vi "Chasis _Omni_Basic.vi"   [LabVIEW 2012, in "Fiel Orientation Compass.lvrbt"]
uses:
  Fiel Orientation Compass.lvrbt
  <vilib>/NXT/Subs/LVHSConnector.ctl
  <vilib>/NXT/NXTIO Xnodes/NXTIOXNode/NXTIO.xnode
  <vilib>/NXT/NXTIO Xnodes/NXTIONodeSubVIs/TETRIX IO Move DC Motors.vi
  <vilib>/NXT/NXTIO Xnodes/AddressXNode/NXTIOAddress.xnode
  <vilib>/FTC/FTC Interpret Motor Power From Left X Axis.vi
  <vilib>/FTC/FTC Interpret Motor Power From Left Y Axis.vi
  <vilib>/FTC/FTC Interpret Motor Power From Right X Axis.vi
  <vilib>/NXT/Dual Mode Library/prims/inRangeAndCoerce/inRangeAndCoerce_int.vi
  <vilib>/NXT/LegoClasses/BrickReference/BrickReference.lvclass
  <vilib>/NXT/Hardware/Plugins/Tetrix DC Motor/TetrixDCMotorAddress.ctl
panel:
  # "This VI was generated based on your configuration in the Remote Control Editor. You may modify the code as needed for your robot. To test this program for an FTC match, return to the Remote Control Editor, select the \"Run Program\" tab, and choose \"FTC Game\"."
types:
  T1 = typedef "LVHSConnector.ctl" = refnum<class "BrickReference.lvclass">
  T2 = typedef "FTC ControllerState.ctl" = cluster{"Left X":i8, "Left Y":i8, "Right X":i8, "Right Y":i8, "Button Encoding 9-12":u8, "Button Encoding 1-8":u8, "POV":T3}
  T3 = typedef "FTC POVState.ctl" = i8
  T4 = typedef "FTC ButtonEventType.ctl" = enum16{"Pressed", "Released"}
  T5 = cluster{"Button ID":enum16{"None", "Button 1", "Button 2", "Button 3", "Button 4", "Button 5", "Button 6", "Button 7", "Button 8", "Button 9", "Button 10", "Button 11", "Button 12", "POV Up", "POV Up Right", "POV Right", "POV Down Right", "POV Down", "POV Down Left", "POV Left", "POV Up Left"}, "Event Type":T4}[]
  T6 = enum16{"None", "Button 1", "Button 2", "Button 3", "Button 4", "Button 5", "Button 6", "Button 7", "Button 8", "Button 9", "Button 10", "Button 11", "Button 12", "POV Up", "POV Up Right", "POV Right", "POV Down Right", "POV Down", "POV Down Left", "POV Left", "POV Up Left"}
  T7 = typedef "TetrixDCMotorAddress.ctl" = i16
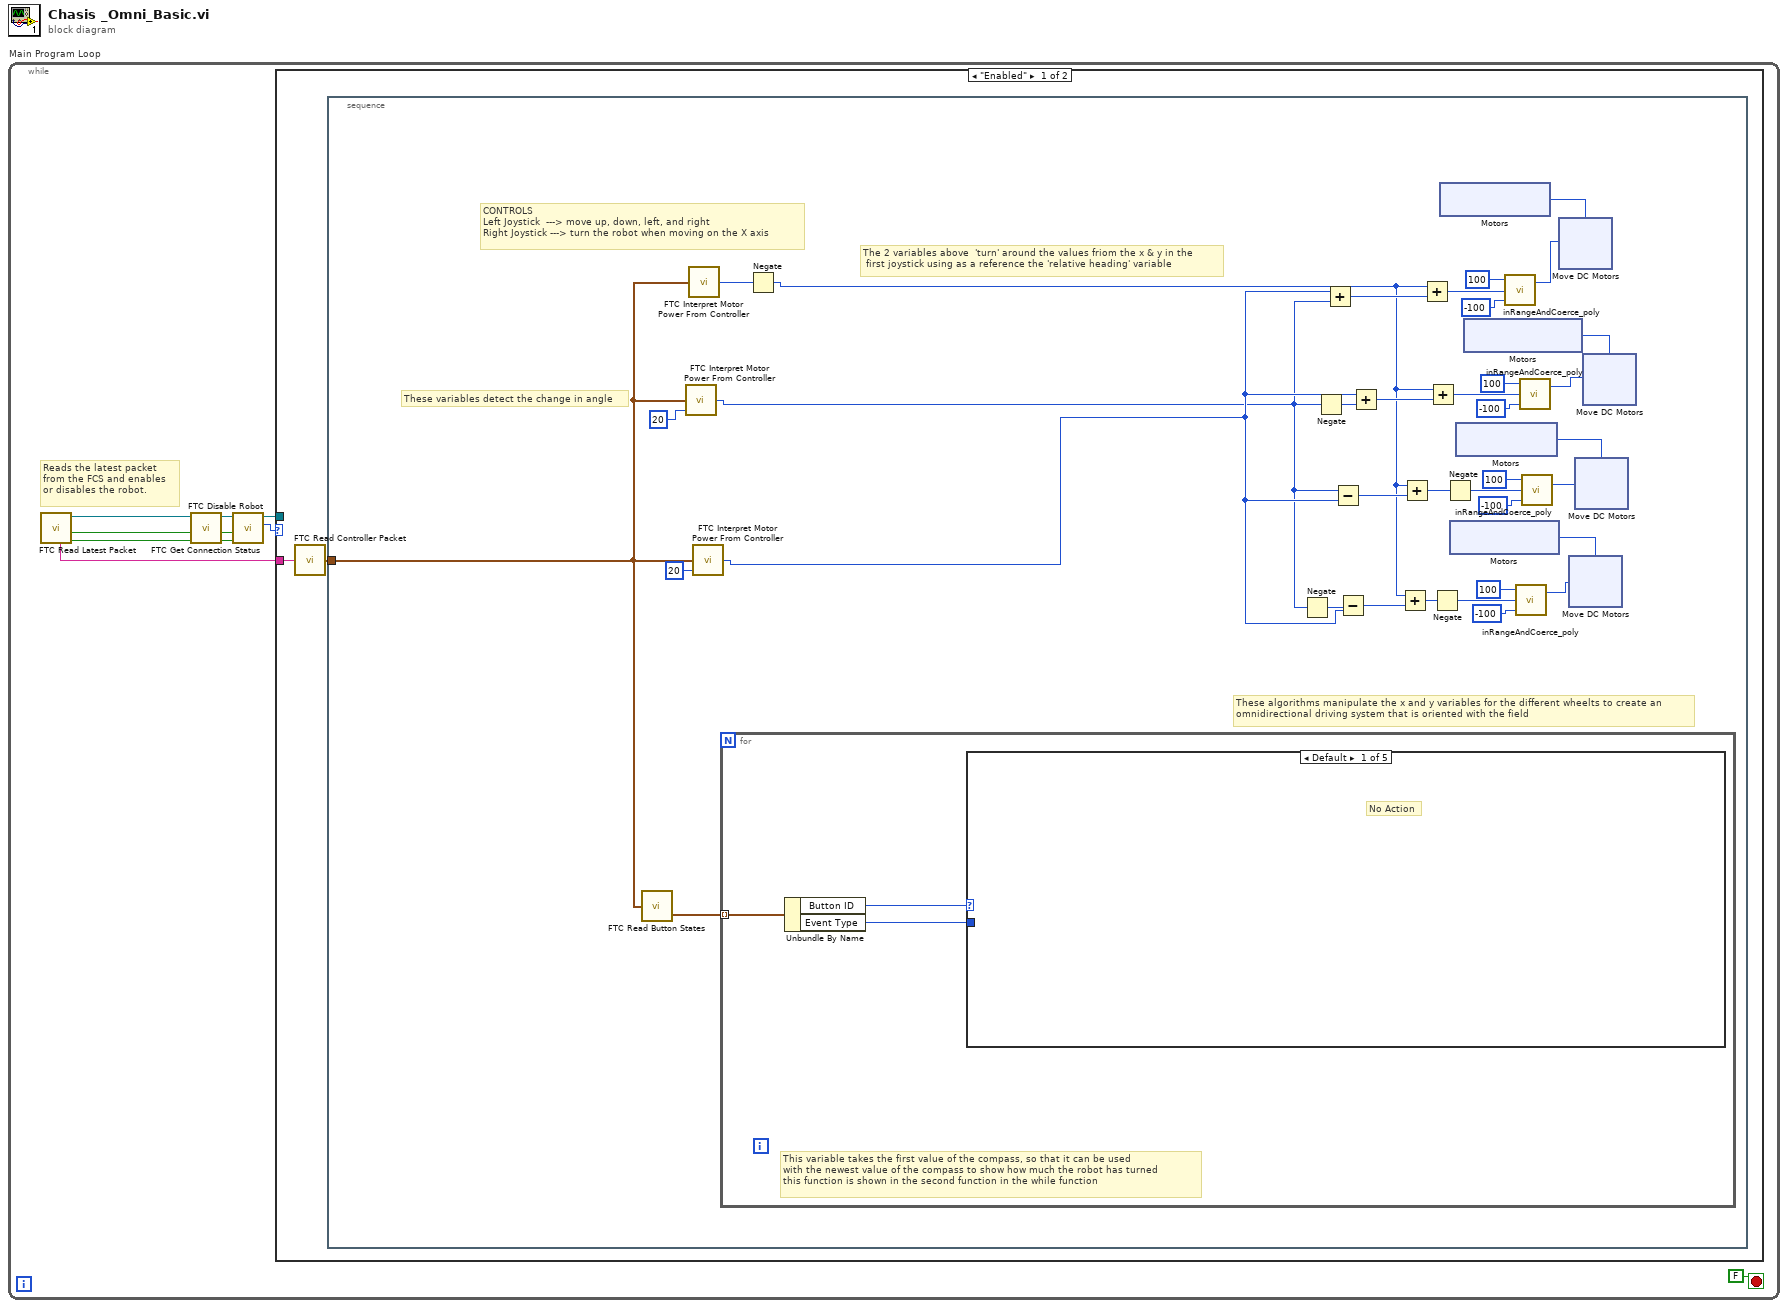
[diagram p0: block diagram]
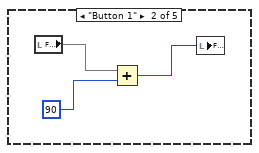
[diagram p2: hidden frame]
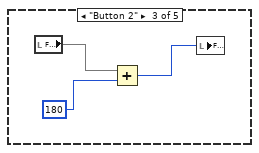
[diagram p3: hidden frame]
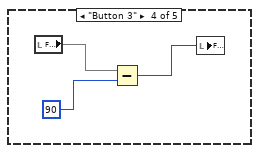
[diagram p4: hidden frame]
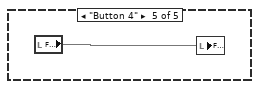
[diagram p5: hidden frame]
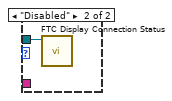
[diagram p6: hidden frame]
diagram:
  n1 = while "Main Program Loop" {
    stop <- FALSE stop-if-true
    # "Reads the latest packet\nfrom the FCS and enables\nor disables the robot."
    n2 = call <vilib>:"FTC Read Latest Packet.vi"() -> ("Packet Received?"=w8:bool, "Stopped?"=w5:bool, "NXT"=w7:T1, "Controller 1"=w9:string)  [unwired: 6 in, 2 out]
    n3 = call <vilib>:"FTC Get Connection Status.vi"("Packet Received?"=w8, "Stopped?"=w5, "NXT"=w7) -> ("Online?"=w2:bool, "Stopped?"=w3:bool, "NXT"=w4:T1)  [unwired: 5 in]
    n4 = call <vilib>:"FTC Disable Robot.vi"("Online?"=w2, "Stopped?"=w3, "NXT"=w4) -> ("Enabled?"=w6:enum16{"Disabled", "Enabled"}, "NXT"=w1:T1)  [unwired: 3 in]
    n5 = case "disableCase" shown="\"Enabled\"" w6 {
      tunnel: w9 -> [w12 _]
      tunnel: w1 -> [_ w94]
      frame "Enabled" {
        n6 = call <vilib>:"FTC Read Controller Packet.vi"("Packet"=w12) -> ("Controller State"=w11:T2)  [unwired: 4 in]
        n7 = stacked-sequence "controller1Actions" {
          tunnel: w11 -> [w48]
          frame #0 {
            # "These algorithms manipulate the x and y variables for the different wheelts to create an\nomnidirectional driving system that is oriented with the field"
            # "The 2 variables above  'turn' around the values friom the x & y in the\n\tfirst joystick using as a reference the 'relative heading' variable"
            # "These variables detect the change in angle"
            # "CONTROLS\nLeft Joystick  ---> move up, down, left, and right                   \nRight Joystick ---> turn the robot when moving on the X axis"
            n8 = call <vilib>:"FTC Read Button States.vi"("Controller State"=w48) -> ("Button Events"=w47:T5)  [unwired: 2 in, 1 out]
            n9 = call-poly <vilib>:"FTC Interpret Motor Power From Controller.vi"("Deadband (10)"=i8 20, "Controller State"=w48) -> ("Power"=w14:i8)  [unwired: 1 in]
            n10 = call-poly <vilib>:"FTC Interpret Motor Power From Controller.vi"("Controller State"=w48) -> ("Power"=w46:i8)  [unwired: 2 in]
            n11 = call-poly <vilib>:"FTC Interpret Motor Power From Controller.vi"("Deadband (10)"=i8 20, "Controller State"=w48) -> ("Power"=w15:i8)  [unwired: 1 in]
            n12 = for "buttonAction" {
              tunnel: w47 -> [w81] mode=indexing
              # "This variable takes the first value of the compass, so that it can be used\nwith the newest value of the compass to show how much the robot has turned \nthis function is shown in the second function in the while function"
              n13 = Unbundle By Name(w81) -> ("Button ID"=w83:T6, "Event Type"=w82:T4)
              n14 = case "EventCase1" shown="Default" w83 {
                tunnel: w82 -> [_ _ _ _ _]
                frame Default {
                  # "No Action"
                }
                frame "Button 1" {
                  n15 = local read item#-1() -> (w86)
                  n16 = Add(x=w86, y=90) -> (x+y=w85:i32)
                  n17 = local write item#-1(w85) -> ()
                }
                frame "Button 2" {
                  n18 = local read item#-1() -> (w89)
                  n19 = Add(x=w89, y=180) -> (x+y=w88:i32)
                  n20 = local write item#-1(w88) -> ()
                }
                frame "Button 3" {
                  n21 = local read item#-1() -> (w92)
                  n22 = Subtract(x=w92, y=90) -> (x-y=w91:i32)
                  n23 = local write item#-1(w91) -> ()
                }
                frame "Button 4" {
                  n24 = local read item#-1() -> (w93)
                  n25 = local write item#-1(w93) -> ()
                }
              }
            }
            n26 = Negate(x=w46) -> (-x=w13:i8)
            n27 = Negate(x=w14) -> (-x=w38:i8)
            n28 = Negate(x=w14) -> (-x=w36:i8)
            n29 = Add(x=w15, y=w14) -> (x+y=w34:i8)
            n30 = Subtract(x=w14, y=w15) -> (x-y=w37:i8)
            n31 = Subtract(x=w38, y=w15) -> (x-y=w39:i8)
            n32 = Add(x=w15, y=w36) -> (x+y=w35:i8)
            n33 = Add(x=w13, y=w39) -> (x+y=w40:i8)
            n34 = Add(x=w13, y=w37) -> (x+y=w41:i8)
            n35 = Add(x=w13, y=w34) -> (x+y=w24:i8)
            n36 = Add(x=w13, y=w35) -> (x+y=w25:i8)
            n37 = Negate(x=w40) -> (-x=w43:i8)
            n38 = xnode "Motors"() -> ("Motor"=w26:T7)
            n39 = Negate(x=w41) -> (-x=w42:i8)
            n40 = xnode "Motors"() -> ("Motor"=w32:T7)
            n41 = xnode "Motors"() -> ("Motor"=w30:T7)
            n42 = xnode "Motors"() -> ("Motor"=w28:T7)
            n43 = call-poly <vilib>:"inRangeAndCoerce_poly.vi"("lower limit"=-100, "x"=w24, "upper limit"=100) -> ("coerced(x)"=w27:i32)  [unwired: 1 out]
            n44 = call-poly <vilib>:"inRangeAndCoerce_poly.vi"("lower limit"=-100, "x"=w43, "upper limit"=100) -> ("coerced(x)"=w33:i32)  [unwired: 1 out]
            n45 = call-poly <vilib>:"inRangeAndCoerce_poly.vi"("lower limit"=-100, "x"=w25, "upper limit"=100) -> ("coerced(x)"=w29:i32)  [unwired: 1 out]
            n46 = call-poly <vilib>:"inRangeAndCoerce_poly.vi"("lower limit"=-100, "x"=w42, "upper limit"=100) -> ("coerced(x)"=w31:i32)  [unwired: 1 out]
            n47 = xnode "Move DC Motors"("Power/Speed 1"=w27, "Motors"=w26) -> ()  [unwired: 1 in, 1 out]
            n48 = xnode "Move DC Motors"("Power/Speed 1"=w33, "Motors"=w32) -> ()  [unwired: 1 in, 1 out]
            n49 = xnode "Move DC Motors"("Power/Speed 1"=w31, "Motors"=w30) -> ()  [unwired: 1 in, 1 out]
            n50 = xnode "Move DC Motors"("Power/Speed 1"=w29, "Motors"=w28) -> ()  [unwired: 1 in, 1 out]
          }
        }
      }
      frame "Disabled" {
        n51 = call <vilib>:"FTC Display Connection Status.vi"("NXT"=w94) -> ()  [unwired: 10 in, 1 out]
      }
    }
  }
